vi "CRYThree Button Dialog CORE.vi"(0 "message":string, 1 "Window Title (\"\")":string, 2 "Justify Message (Left)":enum16{"Left", "Center", "Right"}(ring), 5 "Left Button Text (\"Yes\")":string="Yes", 7 "Right Button Text (\"Cancel\")":string="Cancel", 9 "Center Button Text (\"No\")":string="No", 12 "Keyboard Shortcuts (Left is <Enter>)":T1={"Left Button Key Shortcut"={"Control"=FALSE, "Shift"=FALSE, "Key"="<Enter>"}, "Center Button Key Shortcut"={"Control"=FALSE, "Shift"=FALSE, "Key"=""}, "Right Button Key Shortcut"={"Control"=FALSE, "Shift"=FALSE, "Key"=""}}, 13 "Allow user to close window? (TRUE)":bool=TRUE) -> (4 "Which Button?":T2(ring)=enum."Center Button")   [LabVIEW 2013]
doc: "Displays text in a dialog with three buttons. The output enum indicates which of the three buttons the user chose, or it indicates that the user closed the dialog without making any choice."
panel:
  in  "OK":string="OK"
  out "C-Message":string
  in  "Right Button":bool
  in  "Center Button":bool
  in  "Left Button":bool
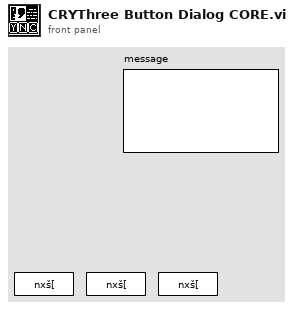
[diagram p1: front panel]
types:
  T1 = cluster{"Left Button Key Shortcut":cluster{"Control":bool, "Shift":bool, "Key":string}, "Center Button Key Shortcut":cluster{"Control":bool, "Shift":bool, "Key":string}, "Right Button Key Shortcut":cluster{"Control":bool, "Shift":bool, "Key":string}}
  T2 = enum16{"Left Button", "Center Button", "Right Button", "Window Close"}
  T3 = cluster{"left":i16, "top":i16, "right":i16, "bottom":i16}
  T4 = cluster{"Control":bool, "Shift":bool, "Key":string}
  T5 = cluster{bool, "Control":bool, "Shift":bool, "Key":string}
  T6 = typedef "LVRectTypeDef.ctl" = cluster{"Left":i16, "Top":i16, "Right":i16, "Bottom":i16}
  T7 = typedef "LVBoundsTypeDef.ctl" = cluster{"Width":u32, "Height":u32}
  T8 = typedef "LVPointTypeDef.ctl" = cluster{"Horizontal":i16, "Vertical":i16}
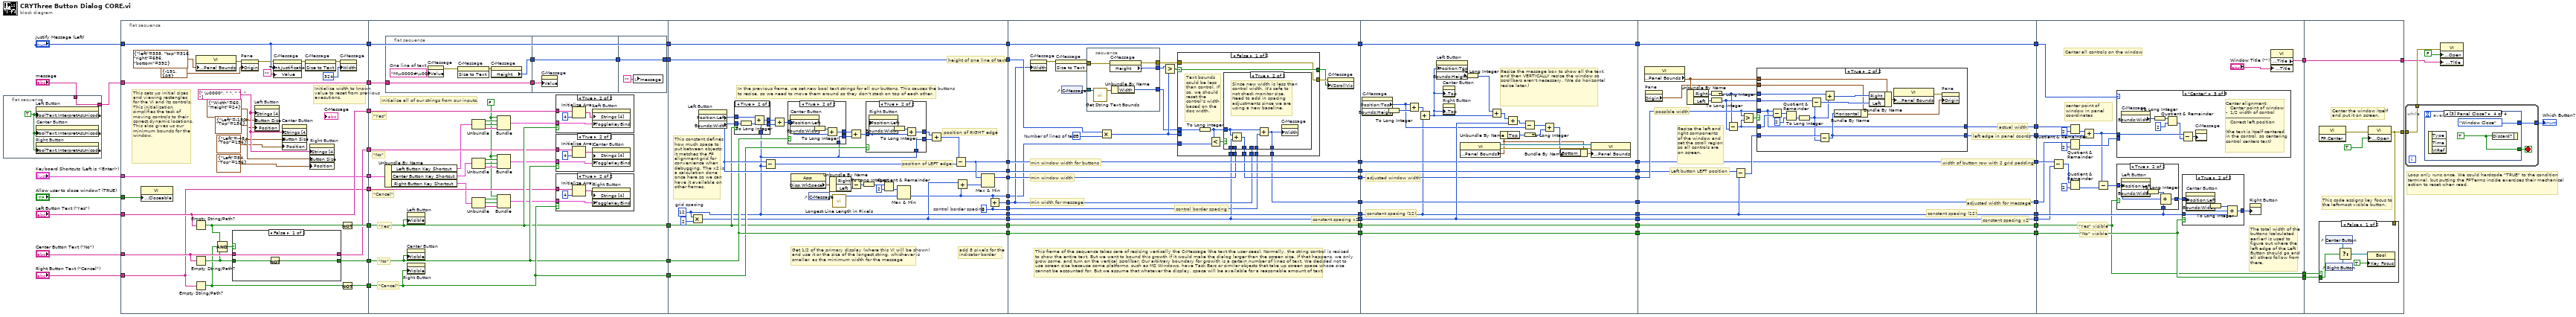
[diagram p0: block diagram]
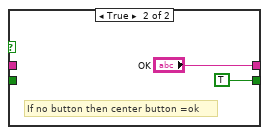
[diagram p2: hidden frame]
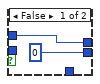
[diagram p6: hidden frame]
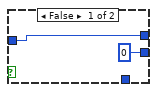
[diagram p7: hidden frame]
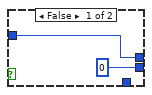
[diagram p8: hidden frame]
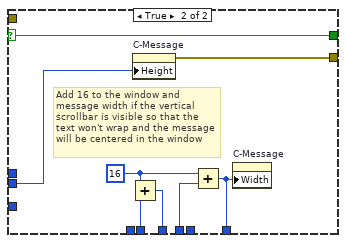
[diagram p10: hidden frame]
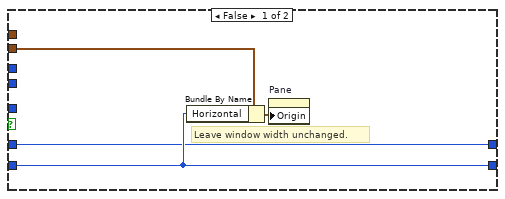
[diagram p11: hidden frame]
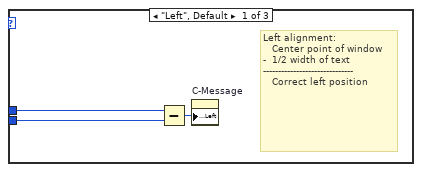
[diagram p12: hidden frame]
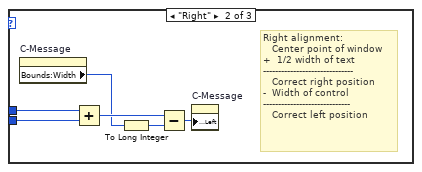
[diagram p13: hidden frame]
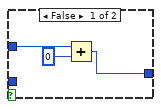
[diagram p14: hidden frame]
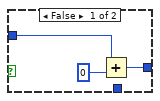
[diagram p15: hidden frame]
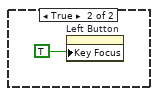
[diagram p16: hidden frame]
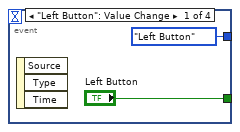
[diagram p17: hidden frame]
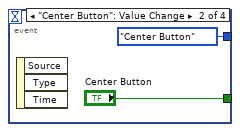
[diagram p18: hidden frame]
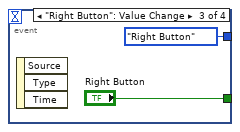
[diagram p19: hidden frame]
diagram:
  # "Loop only runs once. We could hardcode \"TRUE\" to the condition terminal, but putting the FPTerms inside exercises their mechanical action to reset when read."
  n1 = flat-sequence {
    tunnel: "message" -> [w70]
    tunnel: [w70] -> w1
    frame #0 {
      w71 = TRUE ("Boolean Text.Interpret As Unicode")
      n2 = property on="Left Button" class="Bool"("BoolText.InterpretAsUnicode"=w71) -> ()  [unwired: 2 in, 2 out]
      n3 = property on="Center Button" class="Bool"("BoolText.InterpretAsUnicode"=w71) -> ()  [unwired: 2 in, 2 out]
      n4 = property on="Right Button" class="Bool"("BoolText.InterpretAsUnicode"=w71) -> ()  [unwired: 2 in, 2 out]
    }
  }
  n5 = flat-sequence {
    tunnel: [w89] -> w16
    tunnel: [w91] -> w15
    tunnel: [w90] -> w14
    tunnel: [w85] -> w13
    tunnel: [w86] -> w12
    tunnel: [w83] -> w11
    tunnel: [w82] -> w10
    tunnel: "Left Button Text (\"Yes\")" -> [w85]
    tunnel: "Center Button Text (\"No\")" -> [w84]
    tunnel: "Right Button Text (\"Cancel\")" -> [w83]
    tunnel: "Justify Message (Left)" -> [w82]
    tunnel: "Keyboard Shortcuts (Left is <Enter>)" -> [w79]
    tunnel: [w79] -> w9
    tunnel: w1 -> [w78]
    tunnel: [w78] -> w8
    tunnel: "Allow user to close window? (TRUE)" -> [w77]
    tunnel: w16 -> [w133]
    tunnel: [w133] -> w65
    tunnel: w15 -> [w132]
    tunnel: [w132] -> w64
    tunnel: w14 -> [w131]
    tunnel: [w131] -> w63
    tunnel: w13 -> [w130]
    tunnel: w12 -> [w129]
    tunnel: w11 -> [w128]
    tunnel: w10 -> [w127]
    tunnel: [w127] -> w62
    tunnel: [w123] -> w61
    tunnel: w9 -> [w126]
    tunnel: w8 -> [w122]
    tunnel: [w188] -> w60
    tunnel: [w185] -> w59
    tunnel: [w184] -> w58
    tunnel: [w167] -> w57
    tunnel: [w166] -> w56
    tunnel: w65 -> [w177]
    tunnel: w64 -> [w179]
    tunnel: [w179] -> w55
    tunnel: w63 -> [w175]
    tunnel: [w175] -> w54
    tunnel: [w158] -> w53
    tunnel: w62 -> [w170]
    tunnel: [w170] -> w52
    tunnel: w61 -> [w169]
    tunnel: [w169] -> w51
    tunnel: [w156] -> w5
    tunnel: [w155] -> w4
    tunnel: w60 -> [w223]
    tunnel: [w222] -> w50
    tunnel: w59 -> [w229]
    tunnel: [w229] -> w49
    tunnel: w58 -> [w228]
    tunnel: [w228] -> w48
    tunnel: w57 -> [w227]
    tunnel: [w227] -> w47
    tunnel: w56 -> [w216]
    tunnel: [w216] -> w46
    tunnel: w55 -> [w226]
    tunnel: [w226] -> w45
    tunnel: w54 -> [w225]
    tunnel: [w225] -> w44
    tunnel: w53 -> [w217]
    tunnel: [w221] -> w43
    tunnel: w52 -> [w224]
    tunnel: [w224] -> w42
    tunnel: w51 -> [w219]
    tunnel: w5 -> [w215]
    tunnel: w4 -> [w214]
    tunnel: w50 -> [w278]
    tunnel: [w278] -> w41
    tunnel: w49 -> [w277]
    tunnel: [w277] -> w40
    tunnel: w48 -> [w276]
    tunnel: [w276] -> w39
    tunnel: w47 -> [w269]
    tunnel: [w269] -> w38
    tunnel: w46 -> [w286]
    tunnel: [w286] -> w37
    tunnel: w45 -> [w275]
    tunnel: [w275] -> w36
    tunnel: w44 -> [w274]
    tunnel: [w274] -> w35
    tunnel: w43 -> [w273]
    tunnel: [w273] -> w34
    tunnel: w42 -> [w272]
    tunnel: [w272] -> w33
    tunnel: w41 -> [w313]
    tunnel: [w308] -> w32
    tunnel: w40 -> [w301]
    tunnel: [w301] -> w31
    tunnel: w39 -> [w307]
    tunnel: w38 -> [w306]
    tunnel: [w306] -> w30
    tunnel: w37 -> [w300]
    tunnel: [w300] -> w29
    tunnel: [w304] -> w28
    tunnel: w36 -> [w299]
    tunnel: [w299] -> w27
    tunnel: w35 -> [w298]
    tunnel: [w298] -> w26
    tunnel: w34 -> [w295]
    tunnel: [w295] -> w25
    tunnel: w33 -> [w297]
    tunnel: [w297] -> w24
    tunnel: [w338] -> w23
    tunnel: w32 -> [w357]
    tunnel: w31 -> [w350]
    tunnel: w30 -> [w354]
    tunnel: w29 -> [w349]
    tunnel: w28 -> [w356]
    tunnel: w27 -> [w337]
    tunnel: w26 -> [w336]
    tunnel: w25 -> [w342]
    tunnel: w24 -> [w343]
    tunnel: [w337] -> w7
    tunnel: [w336] -> w6
    tunnel: [w391] -> w68
    tunnel: [w393] -> w66
    tunnel: w23 -> [w393]
    tunnel: w7 -> [w389]
    tunnel: w6 -> [w390]
    frame #0 {
      w99 = string[] [" \u0000", " ", " ", " "] ("Strings [4]")
      w98 = cluster{"Width":u32, "Height":u32} {"Width"=60, "Height"=24} ("Button Size")
      # "Initialize width to known value to reset from previous executions."
      # "This sets up initial sizes and viewing rectangles\nfor the VI and its controls. This initialization\nsimplifies the task of moving controls to their\ncorrect dynamic locations. This also gives us our\nminimum bounds for the window."
      n6 = property class="VI"("Front Panel Window:Closeable"=w77) -> ()  [unwired: 2 in, 2 out]
      n7 = Empty String/Path?(string/path=w85) -> (empty?=w93:bool)
      n8 = Empty String/Path?(string/path=w84) -> (empty?=w81:bool)
      n9 = Empty String/Path?(string/path=w83) -> (empty?=w80:bool)
      n10 = property class="VI"("Front Panel Window:Panel Bounds"=T3 {"left"=338, "top"=316, "right"=686, "bottom"=392} ("Front Panel.PanelBounds")) -> (error out=w76:errorcluster)  [unwired: 2 in, 1 out]
      n11 = Compound Arithmetic op=AND(w93, w80, w81) -> (w92:bool)
      n12 = case shown="False" w92 {
        tunnel: w81 -> [w102 _]
        tunnel: [w101 TRUE] -> w91
        tunnel: w84 -> [w100 _]
        tunnel: [w100 "OK"] -> w86
        frame False {
          n13 = Not(x=w102) -> (.not. x?=w101:bool)
        }
        frame True {
          # "If no button then center button =ok"
        }
      }
      n14 = property on="Pane" class="Pane"(error in=w76, "Origin"=cluster{"Horizontal":i16, "Vertical":i16} {"Horizontal"=-191, "Vertical"=109} ("Front Panel.Origin")) -> (error out=w75:errorcluster)  [unwired: 1 in, 1 out]
      n15 = property on="Left Button" class="Bool"("Strings [4]"=w99, "Button Size"=w98, "Position"=cluster{"Left":i32, "Top":i32} {"Left"=-180, "Top"=156}) -> ()  [unwired: 2 in, 2 out]
      n16 = property on="C-Message" class="Str"(error in=w75, "Text.Justification"=w82, "Value"="") -> (error out=w94:errorcluster)  [unwired: 1 in, 1 out]
      n17 = property on="Center Button" class="Bool"("Strings [4]"=w99, "Button Size"=w98, "Position"=cluster{"Left":i32, "Top":i32} {"Left"=-48, "Top"=156}) -> ()  [unwired: 2 in, 2 out]
      n18 = invoke on="C-Message" class="Str" method="Size to Text"(error in=w94) -> (error out=w73:errorcluster)  [unwired: 2 in, 2 out]
      n19 = property on="Right Button" class="Bool"("Strings [4]"=w99, "Button Size"=w98, "Position"=cluster{"Left":i32, "Top":i32} {"Left"=84, "Top"=156}) -> ()  [unwired: 2 in, 2 out]
      n20 = property on="C-Message" class="Str"(error in=w73, "Width"=u32 324 ("Size:Width")) -> ()  [unwired: 1 in, 2 out]
      n21 = Not(x=w93) -> (.not. x?=w90:bool)
      n22 = Not(x=w80) -> (.not. x?=w89:bool)
    }
    frame #1 {
      w107 = FALSE
      # "\"Cancel\""
      # "\"No\""
      # "\"Yes\""
      # "\"Cancel\""
      # "\"No\""
      # "\"Yes\""
      # "Initialize all of our strings from our inputs."
      n23 = Unbundle By Name(w126) -> ("Left Button Key Shortcut"=w120:T4, "Center Button Key Shortcut"=w112:T4, "Right Button Key Shortcut"=w106:T4)
      n24 = flat-sequence {
        tunnel: [w135] -> w125
        tunnel: w122 -> [w134]
        tunnel: [w134] -> w121
        tunnel: w125 -> [w140]
        tunnel: [w140] -> w124
        tunnel: w121 -> [w139]
        tunnel: w124 -> [w141]
        tunnel: [w141] -> w123
        frame #0 {
          w138 = "M\u0000#\u0000,\u0000\"\u0000j\u0000q\u0000A\u0000W\u0000?\u0000>\u0000<\u0000"  # One line of text
          n25 = property on="C-Message" class="Str"("Value"=w138) -> (error out=w136:errorcluster)  [unwired: 2 in, 1 out]
          n26 = invoke on="C-Message" class="Str" method="Size to Text"(error in=w136) -> (error out=w137:errorcluster)  [unwired: 2 in, 2 out]
          n27 = property on="C-Message" class="Str"(error in=w137) -> ("Height"=w135:u32)  [unwired: 1 in, 2 out]
        }
        frame #1 {
          n28 = property on="C-Message" class="Str"("Value"=w139) -> ()  [unwired: 2 in, 2 out]
        }
        frame #2 {
          n29 = local write "message"("") -> ()
        }
      }
      n30 = property on="Left Button" class="Bool"("Visible"=w131) -> ()  [unwired: 2 in, 2 out]
      n31 = property on="Center Button" class="Bool"("Visible"=w132) -> ()  [unwired: 2 in, 2 out]
      n32 = property on="Right Button" class="Bool"("Visible"=w133) -> ()  [unwired: 2 in, 2 out]
      n33 = Unbundle(w120) -> ("Control"=w119:bool, "Shift"=w118:bool, "Key"=w117:string)
      n34 = Unbundle(w112) -> ("Control"=w115:bool, "Shift"=w114:bool, "Key"=w113:string)
      n35 = Unbundle(w106) -> ("Control"=w110:bool, "Shift"=w109:bool, "Key"=w108:string)
      n36 = Bundle(w107, "Control"=w110, "Shift"=w109, "Key"=w108) -> (w105:T5)  [unwired: 1 in]
      n37 = Bundle(w107, "Control"=w119, "Shift"=w118, "Key"=w117) -> (w116:T5)  [unwired: 1 in]
      n38 = Bundle(w107, "Control"=w115, "Shift"=w114, "Key"=w113) -> (w111:T5)  [unwired: 1 in]
      n39 = case shown="True" w131 {
        tunnel: w130 -> [_ w152]
        tunnel: w116 -> [_ w151]
        frame False {
        }
        frame True {
          n40 = Initialize Array(w152, 4 ("dimension size")) -> (w154:string[])
          n41 = property on="Left Button" class="Bool"("Strings [4]"=w154, "ToggleKeyBind"=w151) -> ()  [unwired: 2 in, 2 out]
        }
      }
      n42 = case shown="True" w132 {
        tunnel: w111 -> [_ w148]
        tunnel: w129 -> [_ w147]
        frame False {
        }
        frame True {
          n43 = Initialize Array(w147, 4 ("dimension size")) -> (w150:string[])
          n44 = property on="Center Button" class="Bool"("Strings [4]"=w150, "ToggleKeyBind"=w148) -> ()  [unwired: 2 in, 2 out]
        }
      }
      n45 = case shown="True" w133 {
        tunnel: w105 -> [_ w144]
        tunnel: w128 -> [_ w143]
        frame False {
        }
        frame True {
          n46 = Initialize Array(w143, 4 ("dimension size")) -> (w146:string[])
          n47 = property on="Right Button" class="Bool"("Strings [4]"=w146, "ToggleKeyBind"=w144) -> ()  [unwired: 2 in, 2 out]
        }
      }
    }
    frame #2 {
      w156 = 8  # control border spacing
      w167 = 12  # grid spacing
      # "position of RIGHT edge"
      # "height of one line of text"
      # "add 8 pixels for the indicator border"
      # "Get 1/2 of the primary display (where this VI will be shown) and use it or the size of the longest string, whichever is smaller, as the minimum width for the message"
      # "This constant defines how much space to put between objects; it matches the FP alignment grid for convenience when debugging. The x2 is a calculation done once here so we can have it available on other frames."
      # "In the previous frame, we set new bool text strings for all our buttons. This causes the buttons to resize, so we need to move them around so they don't stack on top of each other."
      # "position of LEFT edge"
      n48 = Multiply(x=w167, y=2) -> (x*y=w166:i32)
      n49 = property on="Left Button" class="Bool"() -> ("Position:Left"=w184:i32, "Bounds:Width"=w181:u32)  [unwired: 2 in, 2 out]
      n50 = case shown="True" w175 {
        tunnel: w184 -> [w191 w196]
        tunnel: w181 -> [_ w195]
        tunnel: [w191 w194] -> w176
        tunnel: w167 -> [_ w192]
        tunnel: [0 w192] -> w174
        frame False {
        }
        frame True {
          n51 = To Long Integer(number=w195) -> (32bit integer=w193:i32)
          n52 = Add(x=w196, y=w193) -> (x+y=w194:i32)
        }
      }
      n53 = Subtract(x=w184, y=w167) -> (x-y=w186:i32)
      n54 = Add(x=w176, y=w174) -> (x+y=w182:i32)
      n55 = case shown="True" w179 {
        tunnel: w182 -> [w205 w210]
        tunnel: [w205 w209] -> w180
        tunnel: [0 w206] -> w173
        tunnel: w167 -> [_ w206]
        frame False {
        }
        frame True {
          n56 = property on="Center Button" class="Bool"("Position:Left"=w210) -> ("Bounds:Width"=w208:u32)  [unwired: 2 in, 2 out]
          n57 = To Long Integer(number=w208) -> (32bit integer=w207:i32)
          n58 = Add(x=w207, y=w210) -> (x+y=w209:i32)
        }
      }
      n59 = property class="App"() -> ("Disp.WkSpace"=w165:T6)  [unwired: 2 in, 2 out]
      n60 = control-ref of="C-Message"() -> (w171:refnum<vi>)
      n61 = Unbundle By Name(w165) -> ("Right"=w161:i16, "Left"=w160:i16)
      n62 = call <vilib>:"Longest Line Length in Pixels.vi"("String"=w171) -> ("longest line length"=w162:i32)  [unwired: 9 in]
      n63 = Add(x=w180, y=w173) -> (x+y=w183:i32)
      n64 = Subtract(x=w161, y=w160) -> (x-y=w164:i16)
      n65 = To Long Integer(number=w164) -> (32bit integer=w159:i32)
      n66 = case shown="True" w177 {
        tunnel: w183 -> [w198 w203]
        tunnel: [w198 w199] -> w178
        tunnel: [0 w200] -> w172
        tunnel: w167 -> [_ w200]
        frame False {
        }
        frame True {
          n67 = property on="Right Button" class="Bool"("Position:Left"=w203) -> ("Bounds:Width"=w202:u32)  [unwired: 2 in, 2 out]
          n68 = To Long Integer(number=w202) -> (32bit integer=w201:i32)
          n69 = Add(x=w201, y=w203) -> (x+y=w199:i32)
        }
      }
      n70 = Quotient & Remainder(x=w159, y=2) -> (floor(x/y)=w157:i32)  [unwired: 1 out]
      n71 = Max & Min(x=w157, y=w162) -> (min(x,y)=w155:i32)  [unwired: 1 out]
      n72 = Add(x=w178, y=w172) -> (x+y=w187:i32)
      n73 = Subtract(x=w187, y=w186) -> (x-y=w185:i32)
      n74 = Add(x=w166, y=w155) -> (x+y=w189:i32)
      n75 = Max & Min(x=w185, y=w189) -> (max(x,y)=w188:i32)  [unwired: 1 out]
      n76 = Add(x=w155, y=w156) -> (x+y=w158:i32)
    }
    frame #3 {
      w231 = u32 25  # Number of lines of text
      # "control border spacing"
      # "constant spacing x2"
      # "min window width for buttons"
      # "min window width"
      # "min width for message"
      # "This frame of the sequence takes care of resizing vertically the C-Message (the text the user sees). Normally, the string control is resized to show the entire text. But we want to bound this growth if it would make the dialog larger than the screen size. If that happens, we only grow some, and turn on the vertical scrollbar. Our arbitrary boundary for growith is a certain number of lines of text. We decided not to use screen size because some platforms, such as MS Windows, have Task Bars or similar objects that take up screen space whose size cannot be accounted for. But we assume that whatever the display, space will be available for a reasonable amount of text."
      n77 = property on="C-Message" class="Str"("Width"=w217) -> (error out=w220:errorcluster)  [unwired: 2 in, 1 out]
      n78 = invoke on="C-Message" class="Str" method="Size to Text"(error in=w220) -> (error out=w235:errorcluster)  [unwired: 2 in, 2 out]
      n79 = control-ref of="C-Message"() -> (w212:refnum<vi>)
      n80 = stacked-sequence {
        tunnel: w235 -> [w241]
        tunnel: [w240] -> w218
        tunnel: [w239] -> w213
        tunnel: w212 -> [w238]
        tunnel: [w236] -> w211
        frame #0 {
          n81 = call <vilib>:"Get String Text Bounds.vi"("String"=w238) -> ("Text bounds"=w237:T7)  [unwired: 10 in]
          n82 = property on="C-Message" class="Str"(error in=w241) -> (error out=w239:errorcluster, "Height"=w240:u32)  [unwired: 1 in, 1 out]
          n83 = Unbundle By Name(w237) -> ("Width"=w236:u32)
        }
      }
      n84 = Multiply(x=w219, y=w231) -> (x*y=w230:u32)
      n85 = Greater?(x=w218, y=w230) -> (0:w234:bool)
      n86 = case shown="False" w234 {
        selector: w234 -> [w253 w267]
        tunnel: [w252 w268] -> w233
        tunnel: [w253 w267] -> w232
        tunnel: w213 -> [w252 _]
        tunnel: w230 -> [_ w266]
        tunnel: [w246 w264] -> w222
        tunnel: w223 -> [w248 w265]
        tunnel: [w245 w261] -> w221
        tunnel: w217 -> [w247 w263]
        tunnel: w211 -> [w250 _]
        tunnel: w214 -> [w249 _]
        tunnel: w216 -> [w244 _]
        tunnel: w215 -> [w243 _]
        frame False {
          # "Text bounds could be less than control. If so, we should reset the control's width based on the doc width."
          n87 = To Long Integer(number=w250) -> (32bit integer=w242:i32)
          n88 = Less?(x=w242, y=w249) -> (x < y?=w251:bool)
          n89 = case shown="True" w251 {
            tunnel: w242 -> [_ w259]
            tunnel: w248 -> [w255 _]
            tunnel: w247 -> [w254 _]
            tunnel: [w255 w258] -> w246
            tunnel: [w254 w256] -> w245
            tunnel: w244 -> [_ w260]
            tunnel: w243 -> [_ w257]
            frame False {
            }
            frame True {
              # "Since new width is less than control width, it's safe to not check monitor size. \nNeed to add in spacing adjustments since we are using a new baseline."
              n90 = Add(x=w259, y=w260) -> (x+y=w258:i32)
              n91 = Add(x=w259, y=w257) -> (x+y=w256:i32)
              n92 = property on="C-Message" class="Str"("Width"=w256) -> ()  [unwired: 2 in, 2 out]
            }
          }
        }
        frame True {
          w262 = 16 ("x")
          # "Add 16 to the window and message width if the vertical scrollbar is visible so that the text won't wrap and the message will be centered in the window"
          n93 = Add(x=w262, y=w265) -> (x+y=w264:i32)
          n94 = property on="C-Message" class="Str"("Height"=w266) -> (error out=w268:errorcluster)  [unwired: 2 in, 1 out]
          n95 = Add(x=w262, y=w263) -> (x+y=w261:i32)
          n96 = property on="C-Message" class="Str"("Width"=w261) -> ()  [unwired: 2 in, 2 out]
        }
      }
      n97 = property on="C-Message" class="Str"(error in=w233, "VScrollVis"=w232) -> ()  [unwired: 1 in, 2 out]
    }
    frame #4 {
      # "adjusted window width"
      # "constant spacing (12)"
      # "Resize the message box to show all the text, and then VERTICALLY resize the window so scrollbars aren't necessary. (We do horizontal resize later.)"
      n98 = property on="C-Message" class="Str"() -> ("Position:Top"=w280:i32, "Bounds:Height"=w279:u32)  [unwired: 2 in, 2 out]
      n99 = To Long Integer(number=w279) -> (32bit integer=w285:i32)
      n100 = Add(x=w280, y=w285) -> (x+y=w270:i32)
      n101 = Add(x=w270, y=w269) -> (x+y=w271:i32)
      n102 = property on="Left Button" class="Bool"("Position:Top"=w271) -> ("Bounds:Height"=w282:u32)  [unwired: 2 in, 2 out]
      n103 = property on="Center Button" class="Bool"("Position:Top"=w271) -> ()  [unwired: 2 in, 2 out]
      n104 = property on="Right Button" class="Bool"("Position:Top"=w271) -> ()  [unwired: 2 in, 2 out]
      n105 = property class="VI"() -> (reference out=w292:refnum<vi>, error out=w293:errorcluster, "Front Panel Window:Panel Bounds"=w283:T6)  [unwired: 2 in]
      n106 = To Long Integer(number=w282) -> (32bit integer=w281:i32)
      n107 = Add(x=w281, y=w271) -> (x+y=w287:i32)
      n108 = Unbundle By Name(w283) -> ("Top"=w290:i16)
      n109 = Add(x=w287, y=w286) -> (x+y=w288:i32)
      n110 = Subtract(x=w288, y=w280) -> (x-y=w291:i32)
      n111 = To Long Integer(number=w290) -> (32bit integer=w284:i32)
      n112 = Add(x=w291, y=w284) -> (x+y=w289:i32)
      n113 = Bundle By Name(cluster=w283, "Bottom"=w289) -> (w294:T6)
      n114 = property class="VI"(reference=w292, error in=w293, "Front Panel Window:Panel Bounds"=w294) -> ()  [unwired: 2 out]
    }
    frame #5 {
      # "adjusted width for message"
      # "constant spacing x2"
      # "constant spacing (12)"
      # "Left button LEFT position"
      # "left edge in panel coords"
      # "width of button row with 2 grid padding"
      # "Resize the left and\nright components\nof the window and\nset the scroll region\nso all controls are \non screen."
      # "actual width"
      # "possible width"
      n115 = property class="VI"() -> ("Front Panel Window:Panel Bounds"=w310:T6)  [unwired: 2 in, 2 out]
      n116 = property on="Pane" class="Pane"() -> ("Origin"=w296:T8)  [unwired: 2 in, 2 out]
      n117 = Unbundle By Name(w310) -> ("Right"=w312:i16, "Left"=w311:i16)
      n118 = To Long Integer(number=w312) -> (32bit integer=w302:i32)
      n119 = To Long Integer(number=w311) -> (32bit integer=w303:i32)
      n120 = Subtract(x=w302, y=w303) -> (x-y=w314:i32)
      n121 = Subtract(x=w307, y=w306) -> (x-y=w305:i32)
      n122 = Greater?(x=w313, y=w314) -> (0:w309:bool)
      n123 = case shown="True" w309 {
        tunnel: w314 -> [w316 w335]
        tunnel: w313 -> [_ w322]
        tunnel: w302 -> [_ w330]
        tunnel: w303 -> [_ w331]
        tunnel: w310 -> [_ w332]
        tunnel: [w318 w324] -> w308
        tunnel: w296 -> [w317 w325]
        tunnel: w305 -> [w318 w323]
        tunnel: [w316 w322] -> w304
        frame False {
          # "Leave window width unchanged."
          n124 = Bundle By Name(cluster=w317, "Horizontal"=w318) -> (w315:T8)
          n125 = property on="Pane" class="Pane"("Origin"=w315) -> ()  [unwired: 2 in, 2 out]
        }
        frame True {
          n126 = Subtract(x=w322, y=w335) -> (x-y=w334:i32)
          n127 = Quotient & Remainder(x=w334, y=2) -> (floor(x/y)=w327:i32)  [unwired: 1 out]
          n128 = To Long Integer(number=w327) -> (32bit integer=w321:i32)
          n129 = Subtract(x=w331, y=w321) -> (x-y=w328:i32)
          n130 = Subtract(x=w323, y=w321) -> (x-y=w324:i32)
          n131 = Add(x=w330, y=w321) -> (x+y=w329:i32)
          n132 = Bundle By Name(cluster=w325, "Horizontal"=w324) -> (w319:T8)
          n133 = Bundle By Name(cluster=w332, "Right"=w329, "Left"=w328) -> (w326:T6)
          n134 = property class="VI"("Front Panel Window:Panel Bounds"=w326) -> (error out=w320:errorcluster)  [unwired: 2 in, 1 out]
          n135 = property on="Pane" class="Pane"(error in=w320, "Origin"=w319) -> ()  [unwired: 1 in, 2 out]
        }
      }
    }
    frame #6 {
      # "\"No\" visible"
      # "\"Yes\" visible"
      # "The total width of the buttons (calculated earlier) is used to figure out where the left edge of the Left Button should go and all others follow from there."
      # "center point of window in panel coordinates"
      # "Center all controls on the window"
      n136 = Subtract(x=w350, y=w349) -> (x-y=w351:i32)
      n137 = Quotient & Remainder(x=w356, y=2) -> (floor(x/y)=w353:i32)  [unwired: 1 out]
      n138 = Quotient & Remainder(x=w342, y=2) -> (floor(x/y)=w341:i32)  [unwired: 1 out]
      n139 = Quotient & Remainder(x=w351, y=2) -> (floor(x/y)=w348:i32)  [unwired: 1 out]
      n140 = Add(x=w353, y=w357) -> (x+y=w340:i32)
      n141 = Subtract(x=w340, y=w348) -> (x-y=w347:i32)
      n142 = case shown="\"Center\"" w343 {
        tunnel: w340 -> [w360 w366 w368]
        tunnel: w341 -> [w358 w365 _]
        frame "Left", Default {
          # "Left alignment:\n   Center point of window\n-  1/2 width of text\n------------------------------\n   Correct left position"
          n143 = Subtract(x=w360, y=w358) -> (x-y=w359:i32)
          n144 = property on="C-Message" class="Str"("Position:Left"=w359) -> ()  [unwired: 2 in, 2 out]
        }
        frame "Right" {
          # "Right alignment:\n   Center point of window\n+  1/2 width of text\n------------------------------\n   Correct right position\n-  Width of control\n-----------------------------\n   Correct left position"
          n145 = property on="C-Message" class="Str"() -> ("Bounds:Width"=w362:u32)  [unwired: 2 in, 2 out]
          n146 = Add(x=w366, y=w365) -> (x+y=w364:i32)
          n147 = To Long Integer(number=w362) -> (32bit integer=w361:i32)
          n148 = Subtract(x=w364, y=w361) -> (x-y=w363:i32)
          n149 = property on="C-Message" class="Str"("Position:Left"=w363) -> ()  [unwired: 2 in, 2 out]
        }
        frame "Center" {
          # "Center alignment:\n   Center point of window\n-  1/2 width of control\n------------------------------\n   Correct left position\n\n(the text is itself centered in the control, so centering control centers text)"
          n150 = property on="C-Message" class="Str"() -> ("Bounds:Width"=w371:u32)  [unwired: 2 in, 2 out]
          n151 = To Long Integer(number=w371) -> (32bit integer=w369:i32)
          n152 = Quotient & Remainder(x=w369, y=2) -> (floor(x/y)=w367:i32)  [unwired: 1 out]
          n153 = Subtract(x=w368, y=w367) -> (x-y=w370:i32)
          n154 = property on="C-Message" class="Str"("Position:Left"=w370) -> ()  [unwired: 2 in, 2 out]
        }
      }
      n155 = case shown="True" w336 {
        tunnel: w354 -> [_ w388]
        tunnel: w347 -> [w383 w387]
        tunnel: [w382 w385] -> w346
        frame False {
          n156 = Add(x=w383, y=0) -> (x+y=w382:i32)
        }
        frame True {
          n157 = property on="Left Button" class="Bool"("Position:Left"=w387) -> ("Bounds:Width"=w386:u32)  [unwired: 2 in, 2 out]
          n158 = To Long Integer(number=w386) -> (32bit integer=w384:i32)
          n159 = Compound Arithmetic op=ADD(w384, w387, w388) -> (w385:i32)
        }
      }
      n160 = case shown="True" w337 {
        tunnel: w354 -> [_ w380]
        tunnel: w346 -> [w375 w378]
        tunnel: [w374 w377] -> w345
        frame False {
          n161 = Add(x=w375, y=0) -> (x+y=w374:i32)
        }
        frame True {
          n162 = property on="Center Button" class="Bool"("Position:Left"=w378) -> ("Bounds:Width"=w379:u32)  [unwired: 2 in, 2 out]
          n163 = To Long Integer(number=w379) -> (32bit integer=w376:i32)
          n164 = Compound Arithmetic op=ADD(w376, w378, w380) -> (w377:i32)
        }
      }
      n165 = property on="Right Button" class="Bool"("Position:Left"=w345) -> ()  [unwired: 2 in, 2 out]
      n166 = property class="VI"("Front Panel Window:Title"="Window Title (\"\")") -> ("Front Panel Window:Title"=w338:string)  [unwired: 2 in, 2 out]
    }
    frame #7 {
      # "This code assigns key focus to\nthe left-most visible button."
      # "Center the window itself and put it on screen."
      n167 = invoke class="VI" method="FP.Center"() -> (error out=w392:errorcluster)  [unwired: 3 in, 2 out]
      n168 = property class="VI"(error in=w392, "Front Panel Window:Open"=TRUE) -> (error out=w391:errorcluster)  [unwired: 1 in, 1 out]
      n169 = case shown="False" w390 {
        tunnel: w391 -> [_ _]
        tunnel: w389 -> [w399 _]
        frame False {
          n170 = control-ref of="Center Button"() -> (w398:refnum<vi>)
          n171 = control-ref of="Right Button"() -> (w397:refnum<vi>)
          n172 = Select(t=w398, s=w399, f=w397) -> (s? t:f=w396:refnum<vi>)
          n173 = property class="Bool"(reference=w396, "Key Focus"=TRUE) -> ()  [unwired: 1 in, 2 out]
        }
        frame True {
          n174 = property on="Left Button" class="Bool"("Key Focus"=TRUE) -> ()  [unwired: 2 in, 2 out]
        }
      }
    }
  }
  n175 = while {
    tunnel: [w403] -> w69
    tunnel: [w402] -> w67
    tunnel: w68 -> [w402]
    stop <- w401 stop-if-true
    n176 = event shown="[3] Panel Close?" {
      selector: _ -> [_ _ _ _]
      dyn-events: _ -> [_ _ _ _]
      timeout: _ -> [_ _ _ _]
      tunnel: ["Left Button" "Center Button" "Right Button" w410] -> w401
      tunnel: [T2."Left Button" ("Which Button?") T2."Center Button" ("Which Button?") T2."Right Button" ("Which Button?") T2."Window Close" ("Which Button?")] -> w403
      event "Left Button": Value Change {
        n177 = event-data() -> ()  [unwired: 1 in, 3 out]
      }
      event "Center Button": Value Change {
        n178 = event-data() -> ()  [unwired: 1 in, 3 out]
      }
      event "Right Button": Value Change {
        n179 = event-data() -> ()  [unwired: 1 in, 3 out]
      }
      event Panel Close? {
        w410 = TRUE ("Discard?")
        n180 = event-data() -> ()  [unwired: 1 in, 3 out]
        n181 = event-data("Discard?"=w410) -> ()  [unwired: 1 in, 1 out]
      }
    }
  }
  "Which Button?" <- w69
  n182 = property class="VI"(error in=w67, "Front Panel Window:Open"=FALSE, "Front Panel Window:Title"=w66) -> ()  [unwired: 1 in, 2 out]
